vi "numeric LV2.vi"(7 "Numeric in":dbl, 11 "Error in":errorcluster, 13 "Operation":T1) -> (8 "Numeric out":dbl, 15 "Error out":errorcluster)   [LabVIEW 2020]
uses:
  Typedefs/operation numeric lv2.ctl
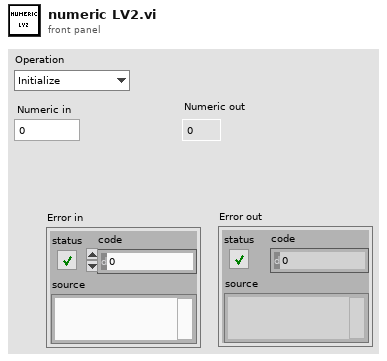
[diagram p1: front panel]
types:
  T1 = typedef "operation numeric lv2.ctl" = enum16{"Initialize", "Read", "Write", ""}
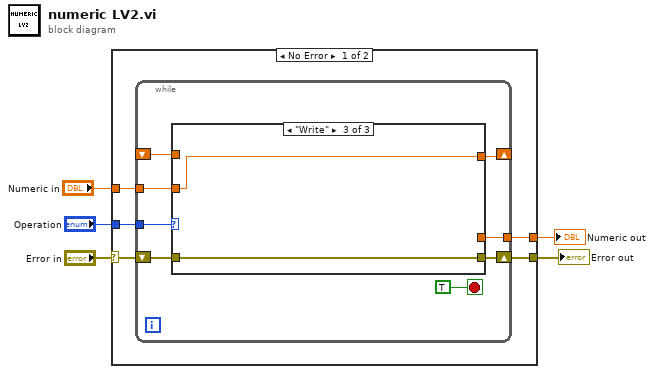
[diagram p0: block diagram]
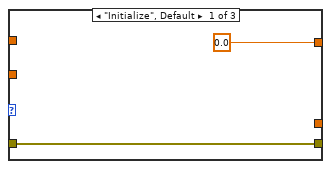
[diagram p2: hidden frame]
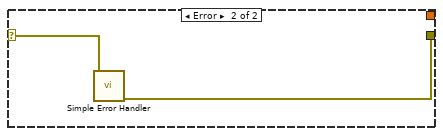
[diagram p4: hidden frame]
diagram:
  n1 = case shown="No Error" "Error in" {
    selector: "Error in" -> [w9 w26]
    tunnel: [w10 w25] -> w4
    tunnel: "Operation" -> [w8 _]
    tunnel: "Numeric in" -> [w7 _]
    tunnel: [w6 _] -> w1
    frame No Error {
      n2 = while {
        shift-right: [w13] -> w10
        shift-left: w9 -> [w12]
        shift-right: [w17] -> _
        shift-left: _ -> [w16]
        tunnel: w8 -> [w18]
        tunnel: w7 -> [w15]
        tunnel: [w14] -> w6
        stop <- TRUE stop-if-true
        n3 = case shown="\"Write\"" w18 {
          tunnel: [0.0 w21 w24] -> w17
          tunnel: w16 -> [_ w21 _]
          tunnel: w15 -> [_ _ w24]
          tunnel: [_ w21 _] -> w14
          tunnel: [w19 w22 w23] -> w13
          tunnel: w12 -> [w19 w22 w23]
          frame "Initialize", Default {
          }
          frame "Read" {
          }
          frame "Write" {
          }
        }
      }
    }
    frame Error {
      n4 = call <vilib>:"Simple Error Handler.vi"("error in (no error)"=w26) -> ("error out"=w25:errorcluster)  [unwired: 4 in, 4 out]
    }
  }
  "Error out" <- w4
  "Numeric out" <- w1
